vi "P2022 TB INCAR.vi"() -> ()   [LabVIEW 2013]
doc: "Use this template to build a producer/consumer design pattern with events to produce queue items. Use this design pattern instead of the user interface event handler pattern for user interfaces when you want to execute code asynchronously in response to an event without slowing the user interface responsiveness."
uses:
  Controles/P2022 Datos Control.ctl
  Controles/P2018 Com Control.ctl
  serialBronkhorst/_s_TablaBronkhorst.ctl
  Controles/P2018 Arduino Control.ctl
  Controles/Functions.ctl
  Controles/User Event Data.ctl
  Controles/Data Type.ctl
  Controles/Change Control.ctl
  Controles/PassedVars.ctl
  P2022 TB INCAR GLOBALES.vi
panel:
  out "ESTADO":T1
  out "SP_EXTRA":dbl format="%.1f"
  out "mst0":i32
  out "mst1":i32
  in  "Tab Control":T2(tab)
  out "String1f":string
  out "String2f":string
  out "String3f":string
  out "String4f":string
  out "FLUJO8":dbl caption="ln/h" format="%.2f"
  out "FLUJO7":dbl caption="ln/h" format="%.2f"
  out "FLUJO6":dbl caption="ln/h" format="%.2f"
  out "FLUJO5":dbl caption="ln/h" format="%.2f"
  out "Lvalve":bool
  out "Lflujo4":bool
  out "Lflujo3":bool
  out "Lflujo2":bool
  out "Lflujo1":bool
  in  "Modulo":u32=1 max=1000 step=1
  in  "Comments":string="Añade aqui los comentarios...... y pincha fuera (sin teclear ENTER)"
  out "TEMP_EXTRA":dbl format="%.1f"
  out "TEMP_CINTA":dbl format="%.1f"
  out "SP_CINTA":dbl format="%.1f"
  out "TEMP_INF":dbl format="%.1f"
  out "SP_TINF":dbl format="%.1f"
  out "TEMP_SUP":dbl format="%.1f"
  out "SP_TSUP":dbl format="%.1f"
  out "TIEMPO(min)":dbl format="%.2f"
  out "PESO(mg)":dbl format="%.1f"
  out "TEMPERATURA(C)":dbl format="%.1f"
  out "FLUJO4":dbl caption="ln/h" format="%.2f"
  out "FLUJO3":dbl caption="ln/h" format="%.2f"
  out "FLUJO2":dbl caption="ln/h" format="%.2f"
  out "FLUJO1":dbl caption="g/h" format="%.2f"
  out "Sampling(ms)":i32
  out "Lsample":bool
  out "Estado":string
  in  "Calibrar":bool
  in  "Muestreo":bool
  in  "Temperatura":bool
  in  "Programar":bool
  in  "Fin":bool
  in  "Auto":bool
  in  "Manual":bool
  in  "Reles":bool
  in  "Flujos":bool
  in  "Parar":bool
  out "String1s":string
  out "String2s":string
  out "String3s":string
  out "String4s":string
  out "Tempex(C),":dbl format="%.1f"
  out "XY Peso":cluster{dbl[], dbl[]}[](graph)
  out "Tiempo(min),":dbl format="%.2f"
  out "Pesotb(mg),":dbl format="%.2f"
  out "Temptb(C),":dbl format="%.1f"
  out "Ttermob(C)":dbl format="%.1f"
  out "XYTemp":cluster{dbl[], dbl[]}[](graph)
  out "Tsuperior(C)":dbl format="%.1f"
  out "Tinferior(C)":dbl format="%.1f"
  out "TcintaC)":dbl format="%.1f"
  out "Textra(C)":dbl format="%.1f"
  out "XYTemPes":cluster{dbl[], dbl[]}(graph)
  out "Temptb(C)_":dbl format="%.1f"
  out "Pesotb(mg)_":dbl format="%.2f"
  out "Flujo8.":dbl format="%.2f"
  out "Flujo7.":dbl format="%.2f"
  out "Flujo6.":dbl format="%.2f"
  out "Flujo5.":dbl format="%.2f"
  out "XYFlows":cluster{dbl[], dbl[]}[](graph)
  out "Flujo4.":dbl format="%.2f"
  out "Flujo3.":dbl format="%.2f"
  out "Flujo2.":dbl format="%.2f"
  out "Flujo1.":dbl format="%.2f"
  in  "Completa":i32(listbox)
  in  "Secuencia":bool
  in  "Reducida":i32(listbox)
  in  "Pausa":bool
  in  "Saltar":bool
  in  "Max_t (s)":dbl=900.0 min=0.0 max=999.9 step=0.1 format="%.1f"
  in  "Delta_t (s)":dbl=60.0 min=0.0 max=999.9 step=0.1 format="%.1f"
  in  "Delta_T (C)":dbl=1.0 min=0.0 max=999.9 step=0.1 format="%.1f"
  out "PASOS":string[](array[string])
  out "FLOWBUS MassFlowDevs":T3
  out "SERIAL MassFlowDevs":T3
  out "Datos":T4 {"fFSET4" format="%#.6f"; "fFSET3" format="%#.6f"; "fFSET2" format="%#.6f"; "fFSET1" format="%#.6f"; "fFLUJO4" format="%#.6f"; "fFLUJO2" format="%#.6f"; "fFLUJO1" format="%#.6f"; "fFLUJO3" format="%#.6f"; "T_EXTRA" format="%#.6f"; "TSET_EXTRA" format="%#.6f"; "T_CINTA" format="%#.6f"; "TSET_CINTA" format="%#.6f"; "sFSET4" format="%#.6f"; "POSICION" format="%#.6f"; "TEMP_SUP" format="%#.6f"; "TSET_SUP" format="%#.6f"; "PESO_TB" format="%#.6f"; "TEMP_TB" format="%#.6f"; "TEMP_INF" format="%#.6f"; "sFSET3" format="%#.6f"; "sFSET2" format="%#.6f"; "sFSET1" format="%#.6f"; "V_VAPOR" format="%#.6f"; "sFLUJO4" format="%#.6f"; "sFLUJO2" format="%#.6f"; "sFLUJO1" format="%#.6f"; "TSET_INF" format="%#.6f"; "TIEMPO" format="%#.6f"; "sFLUJO3" format="%#.6f"}
  out "error out":errorcluster
  out "Comunicaciones":T5={"Flujo_1"="ASRL6::INSTR", "Brk1"=FALSE, "Flujo_2"="ASRL6::INSTR", "Brk2"=FALSE, "Flujo_3"="ASRL6::INSTR", "Brk3"=FALSE, "Flujo_4"="ASRL6::INSTR", "Brk4"=FALSE, "Eurothe"="ASRL6::INSTR", "Eurot"=FALSE, "Balanza"="ASRL6::INSTR", "Bal"=FALSE, "eValPos"="ASRL6::INSTR", "eVal"=FALSE, "flowbus"="ASRL6::INSTR", "fb"=FALSE}
  out "PESO":string
  out "TEMPERATURA":string
  out "Array":dbl[][](array[numeric])
  in  "Secuencia":string[](array[string])
  # "INCAR  TB \nEnero 2023 Ver2.3.1"
  # "a-sslcdms 01/2023"
  # "Termobalanza      ___________________________________"
  # "Horno y cinta"
  # "Temperatura extra"
  # "Termobalanza"
  # "Termobalanza      ___________________________"
  # "SERIE                          Controladores de flujo                     FLOWBUS"
  # "Condiciones de estabilidad en temperatura"
  # "Maxima variación \nde temperatura"
  # "en este intervalo \nde tiempo."
  # "Maximo tiempo posible \nsin alcanzar estabilidad"
  # "TERMOBALANZA"
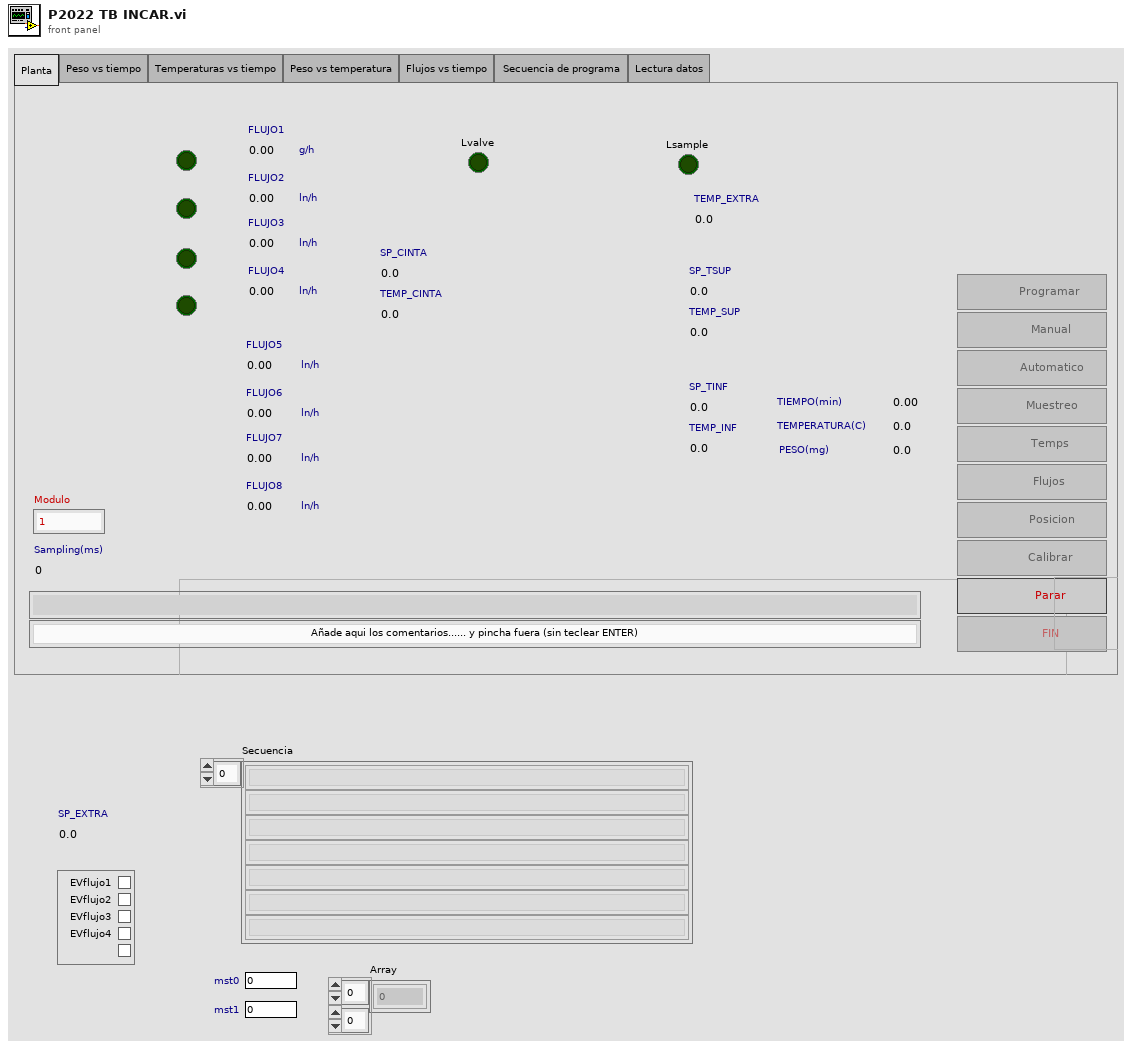
[diagram p1: front panel]
types:
  T1 = typedef "P2018 Arduino Control.ctl" = cluster{"EVflujo1":bool, "EVflujo2":bool, "EVflujo3":bool, "EVflujo4":bool, "Evalve":bool}
  T2 = enum32{"Planta", "Peso vs tiempo", "Temperaturas vs tiempo", "Peso vs temperatura", "Flujos vs tiempo", "Secuencia de programa ", "Lectura datos"}
  T3 = typedef "_s_TablaBronkhorst.ctl" = string[][]
  T4 = typedef "P2022 Datos Control.ctl" = cluster{"TIEMPO":dbl, "sFSET1":dbl, "sFLUJO1":dbl, "sFSET2":dbl, "sFLUJO2":dbl, "sFSET3":dbl, "sFLUJO3":dbl, "sFSET4":dbl, "sFLUJO4":dbl, "TSET_SUP":dbl, "TEMP_SUP":dbl, "TSET_INF":dbl, "TEMP_INF":dbl, "TSET_CINTA":dbl, "T_CINTA":dbl, "TSET_EXTRA":dbl, "T_EXTRA":dbl, "TEMP_TB":dbl, "PESO_TB":dbl, "POSICION":dbl, "V_VAPOR":dbl, "fFSET1":dbl, "fFLUJO1":dbl, "fFSET2":dbl, "fFLUJO2":dbl, "fFSET3":dbl, "fFLUJO3":dbl, "fFSET4":dbl, "fFLUJO4":dbl}
  T5 = typedef "P2018 Com Control.ctl" = cluster{"Flujo_1":refnum<visa-resource-name>, "Brk1":bool, "Flujo_2":refnum<visa-resource-name>, "Brk2":bool, "Flujo_3":refnum<visa-resource-name>, "Brk3":bool, "Flujo_4":refnum<visa-resource-name>, "Brk4":bool, "Eurothe":refnum<visa-resource-name>, "Eurot":bool, "Balanza":refnum<visa-resource-name>, "Bal":bool, "eValPos":refnum<visa-resource-name>, "eVal":bool, "flowbus":refnum<visa-resource-name>, "fb":bool}
  T6 = enum32{"Planta", "Peso vs tiempo", "Temperaturas vs tiempo", "Peso vs temperatura", "Flujos vs tiempo", "Secuencia de programa "}
  T7 = typedef "User Event Data.ctl" = cluster{"Data Type":T8, "Data":variant}
  T8 = typedef "Data Type.ctl" = enum16{"Init FP", "En/Dis FP Ctls", "Update FP", "Upd Status", "Upd Seq"}
  T9 = typedef "Functions.ctl" = enum16{"Initialize", "Run Man", "Run Auto", "Stop"}
  T10 = typedef "Change Control.ctl" = enum16{"Default", "Continue", "Change Flows", "Change Valves", "Change Temp"}
  T11 = typedef "PassedVars.ctl" = dbl
  T12 = typedef "P2018 Bronkhorst Control.ctl" = cluster{"Dispositivos":T3, "NuevosSP":string[][], "Nodes":u32, "Delay(s)":dbl}
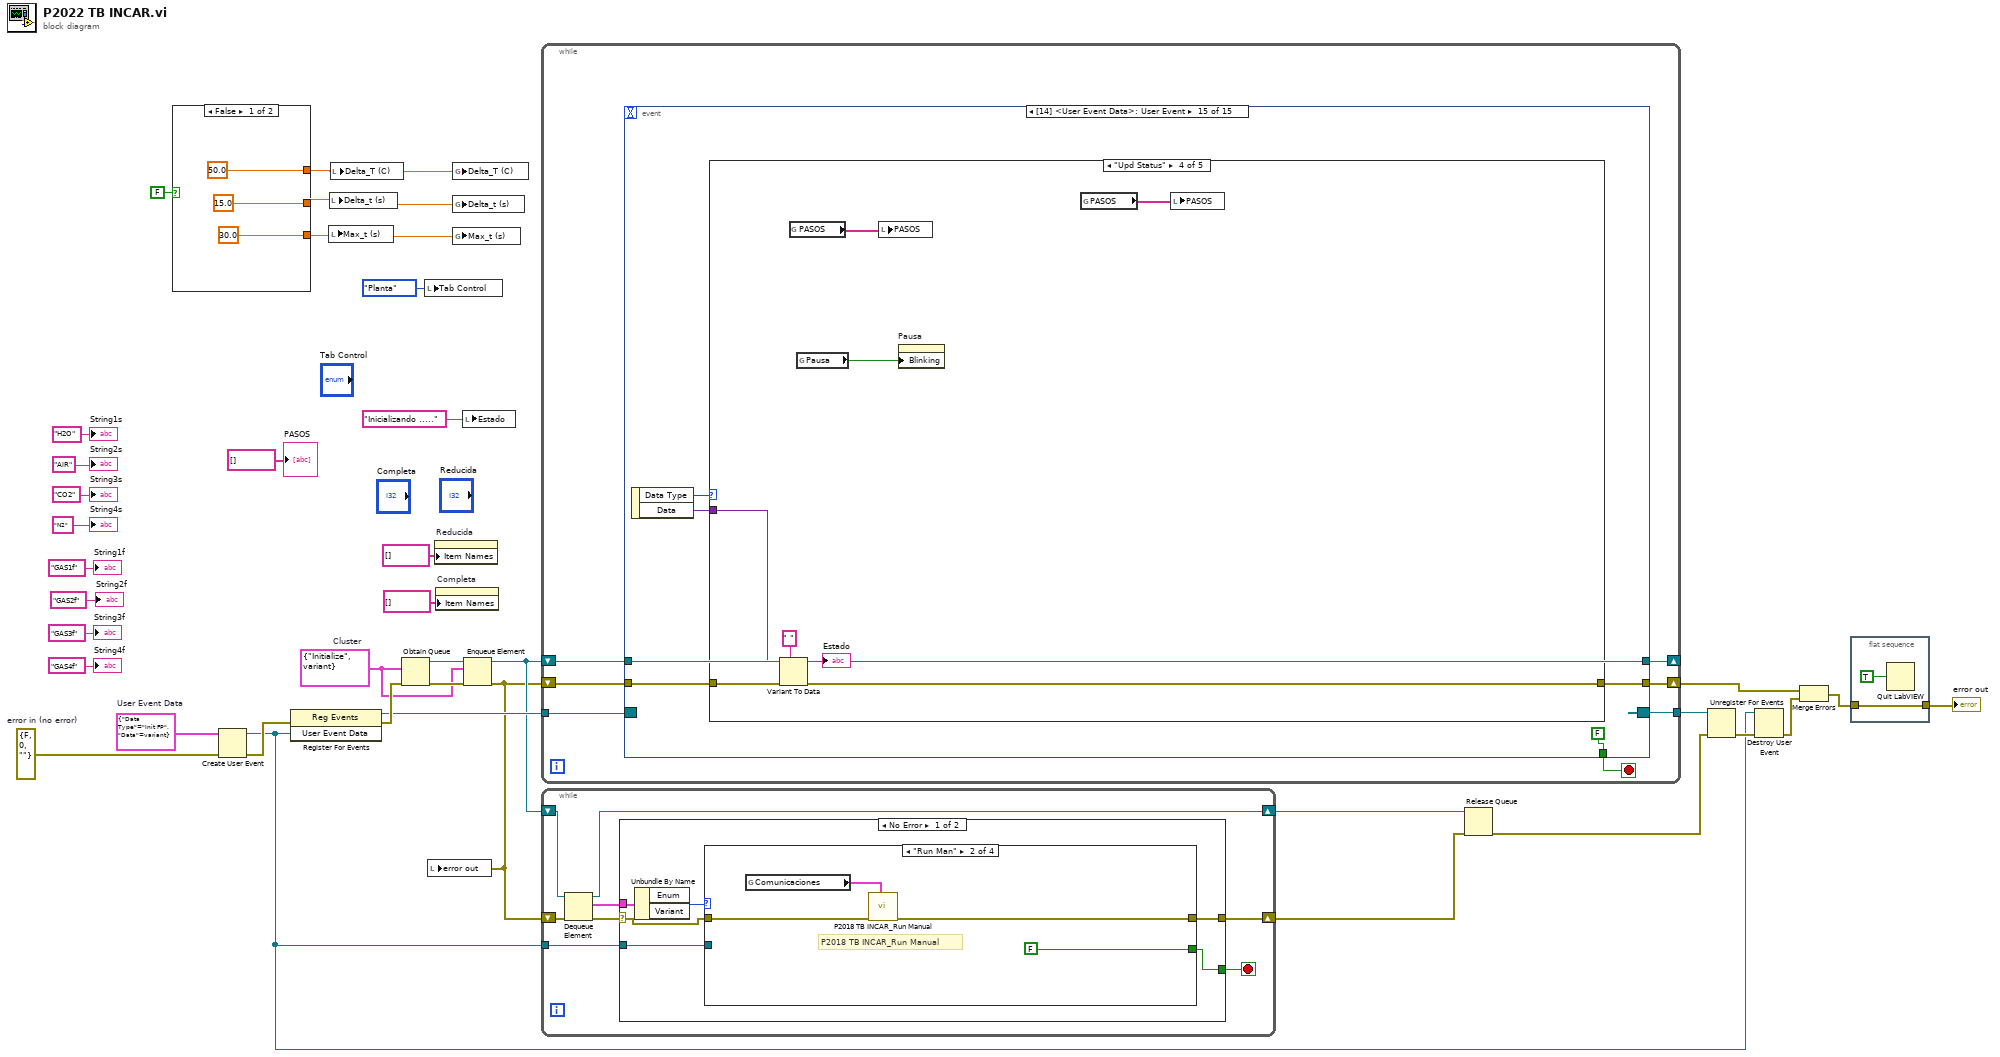
[diagram p0: block diagram]
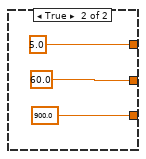
[diagram p2: hidden frame]
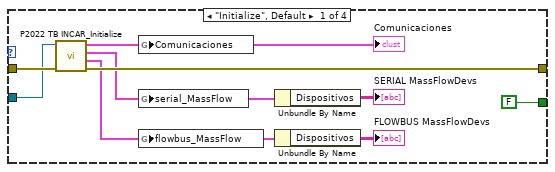
[diagram p3: hidden frame]
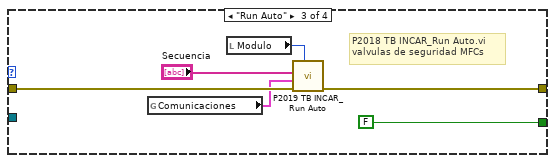
[diagram p4: hidden frame]
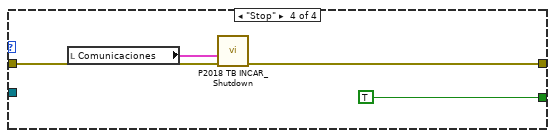
[diagram p5: hidden frame]
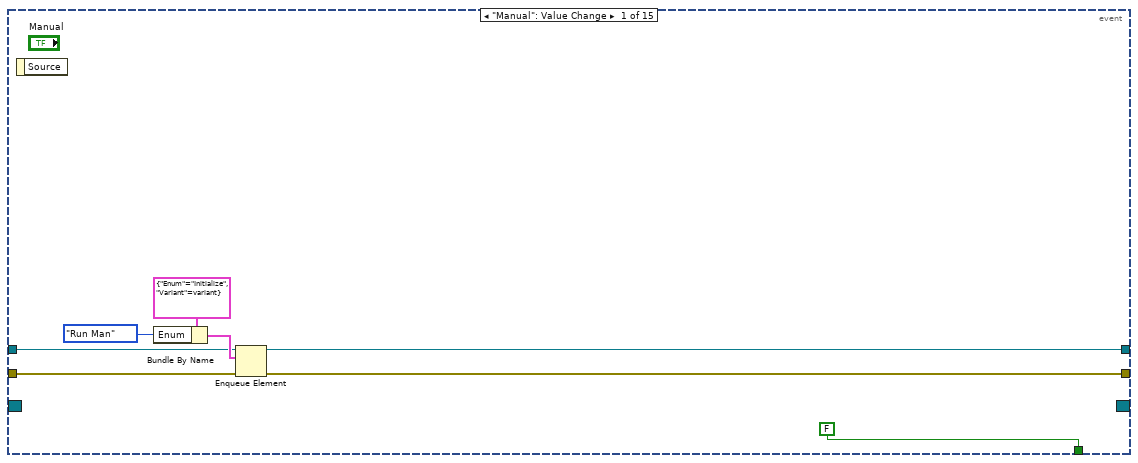
[diagram p7: hidden frame]
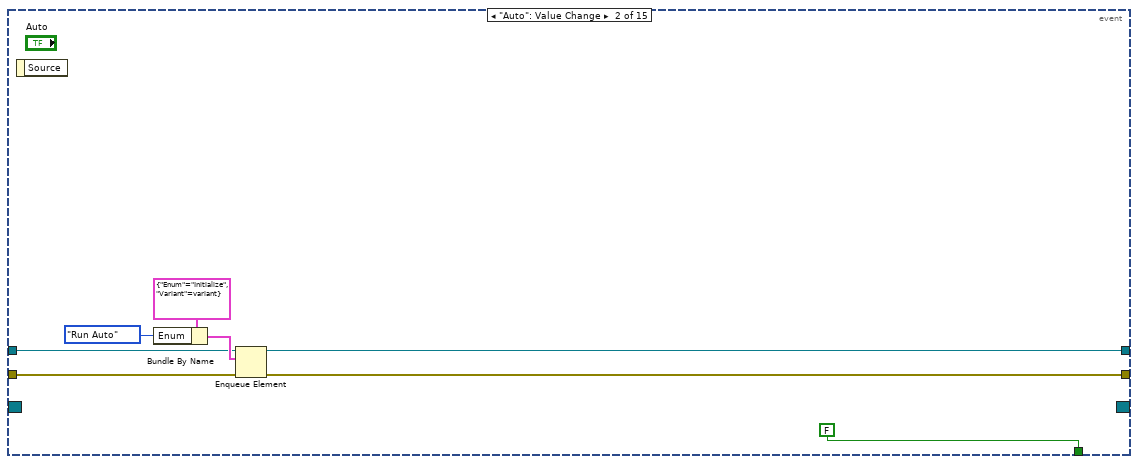
[diagram p8: hidden frame]
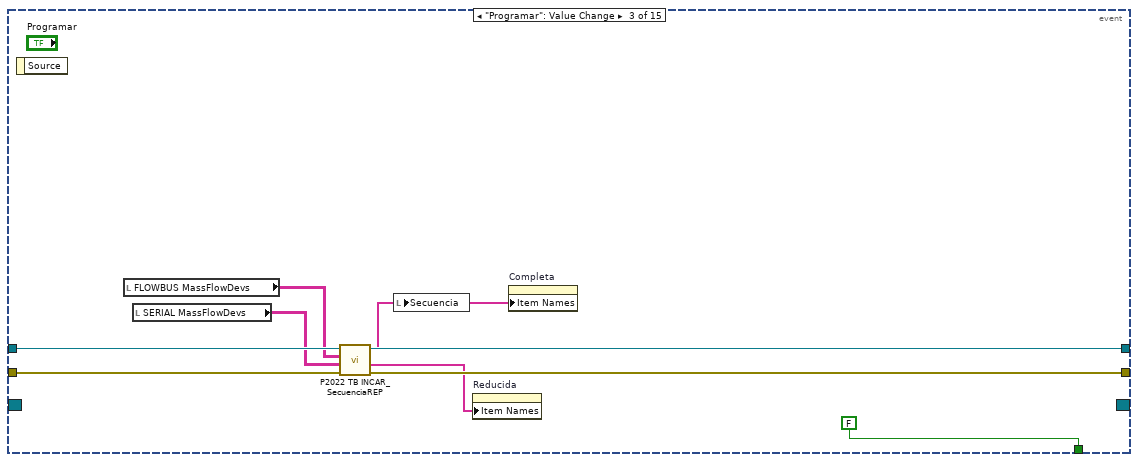
[diagram p9: hidden frame]
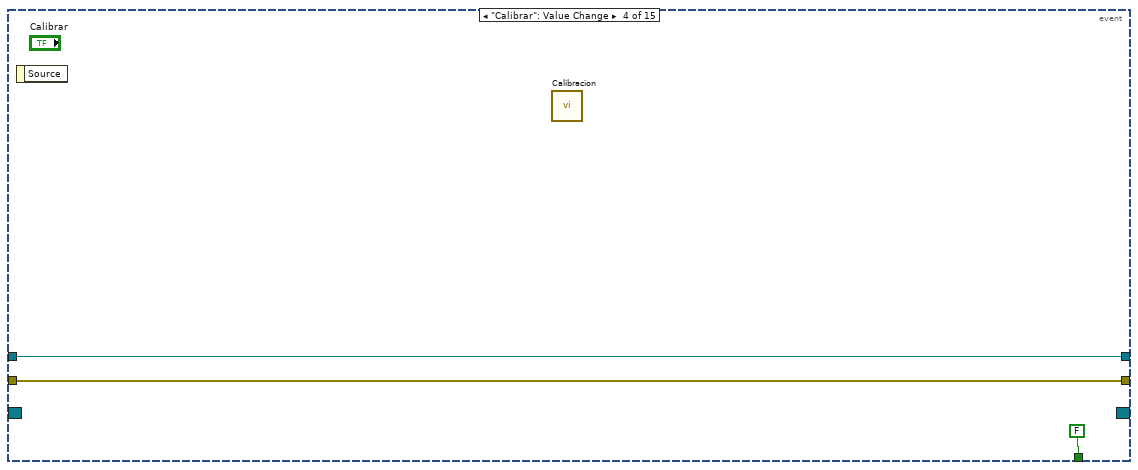
[diagram p10: hidden frame]
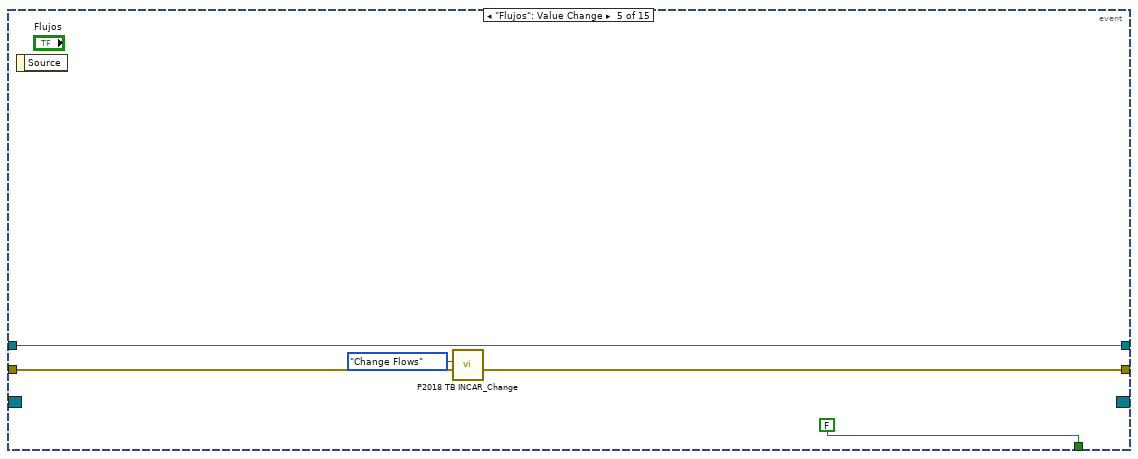
[diagram p11: hidden frame]
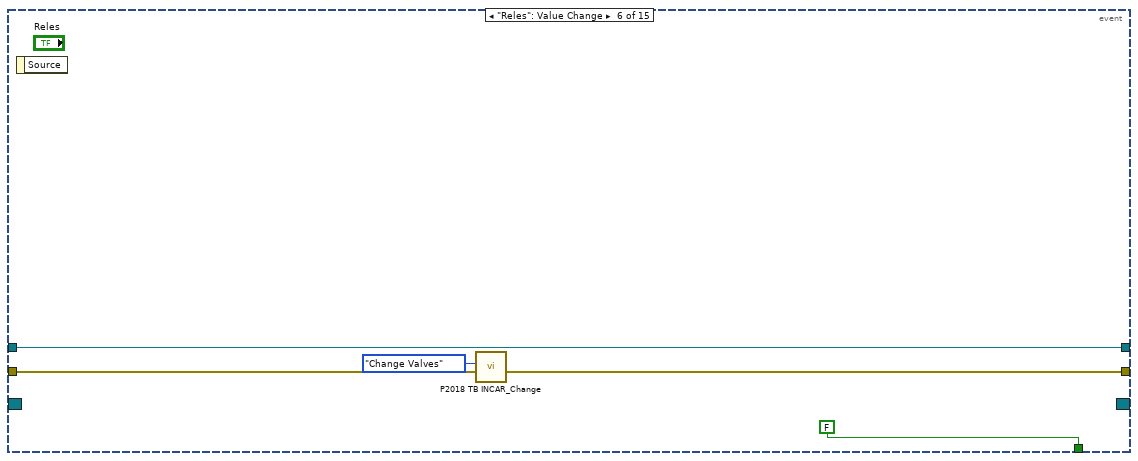
[diagram p12: hidden frame]
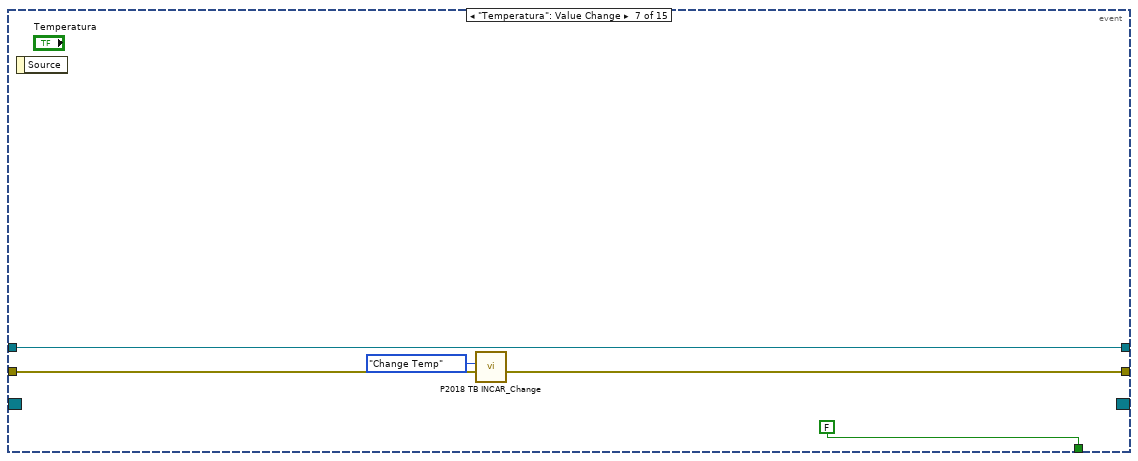
[diagram p13: hidden frame]
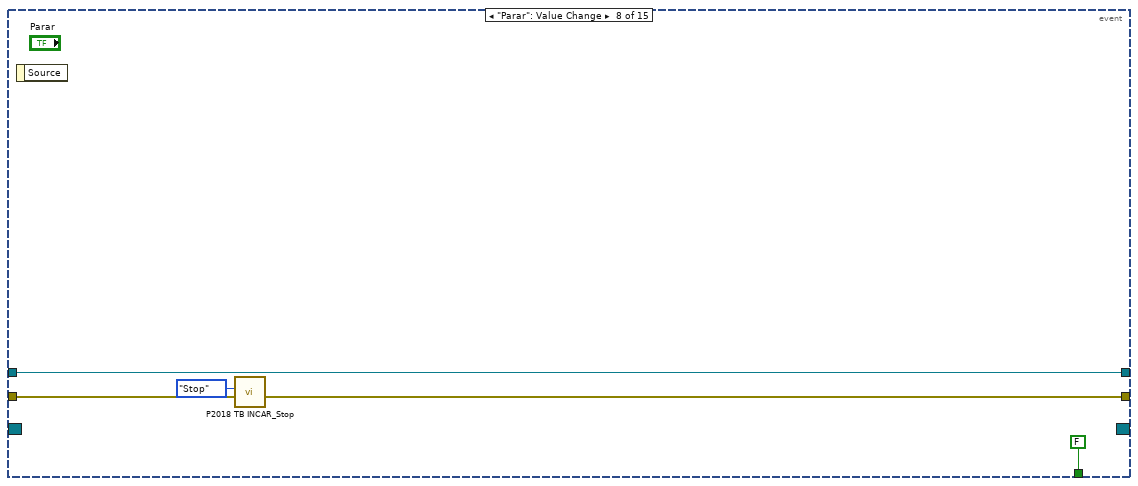
[diagram p14: hidden frame]
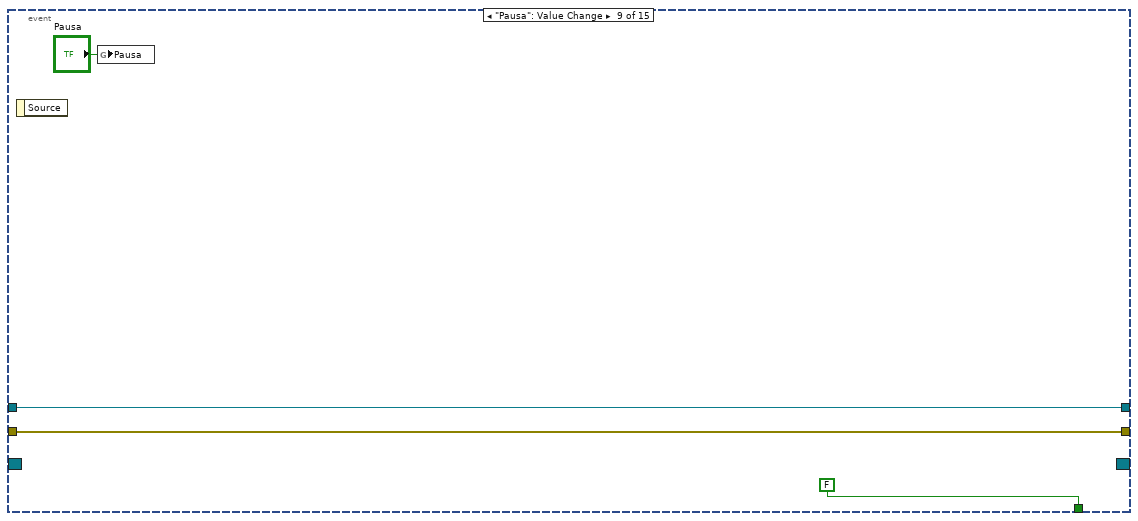
[diagram p15: hidden frame]
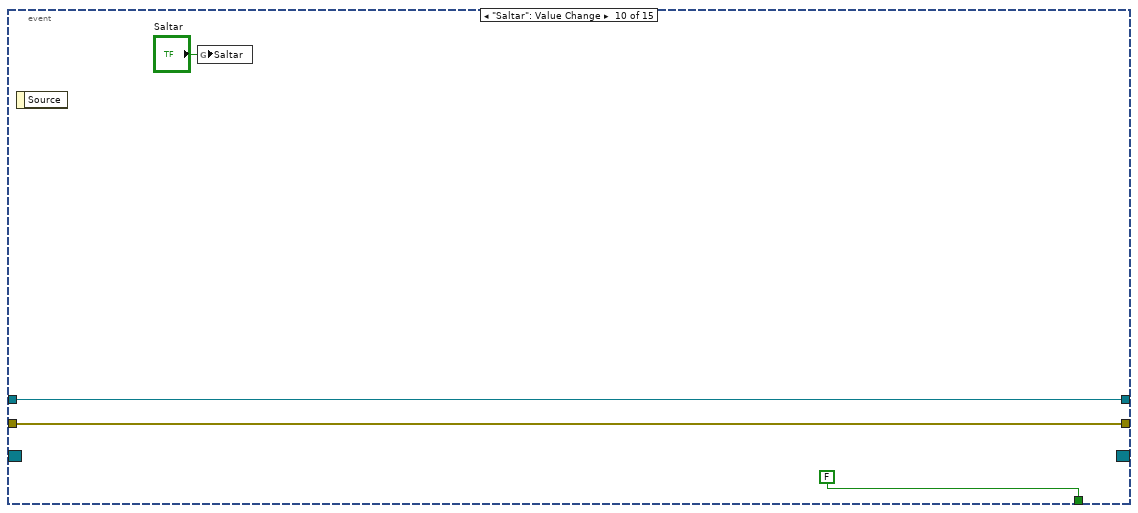
[diagram p16: hidden frame]
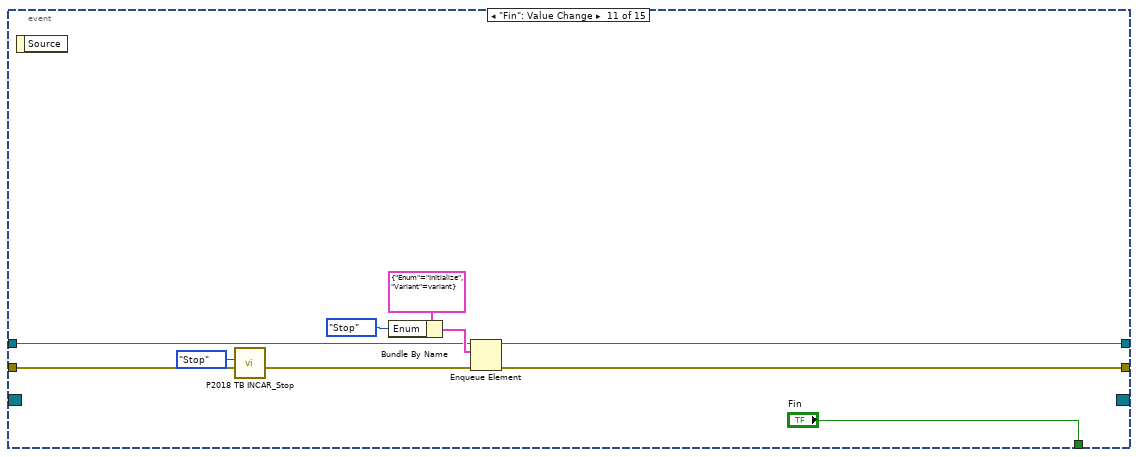
[diagram p17: hidden frame]
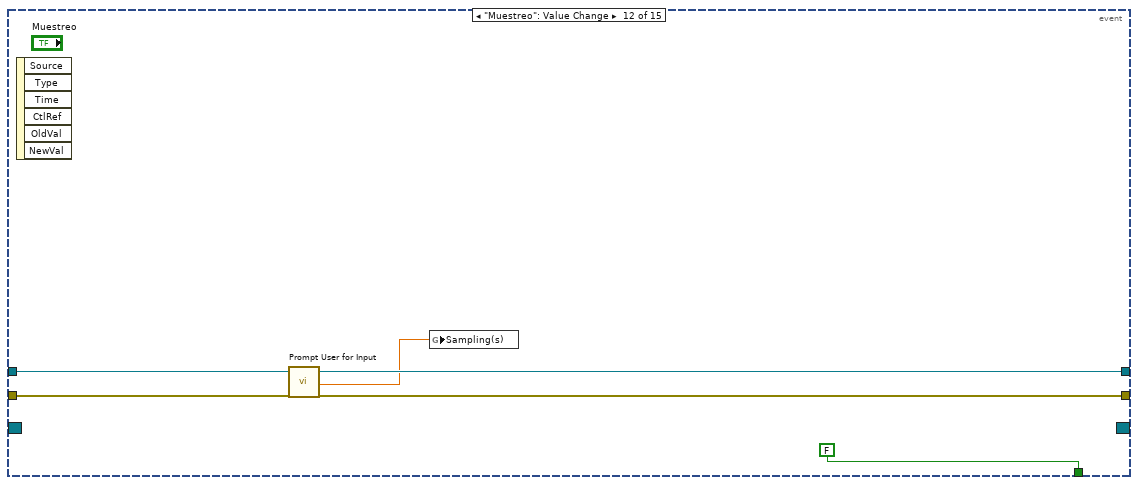
[diagram p18: hidden frame]
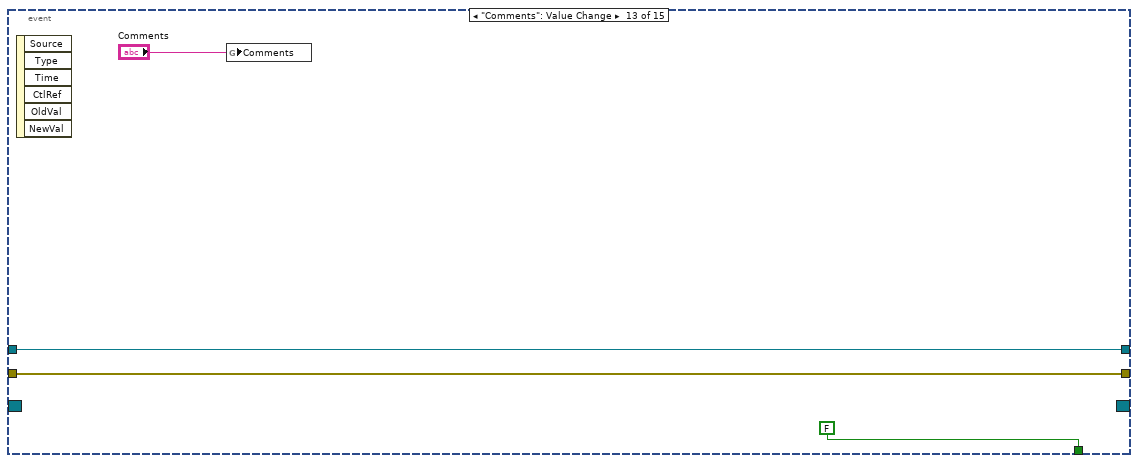
[diagram p19: hidden frame]
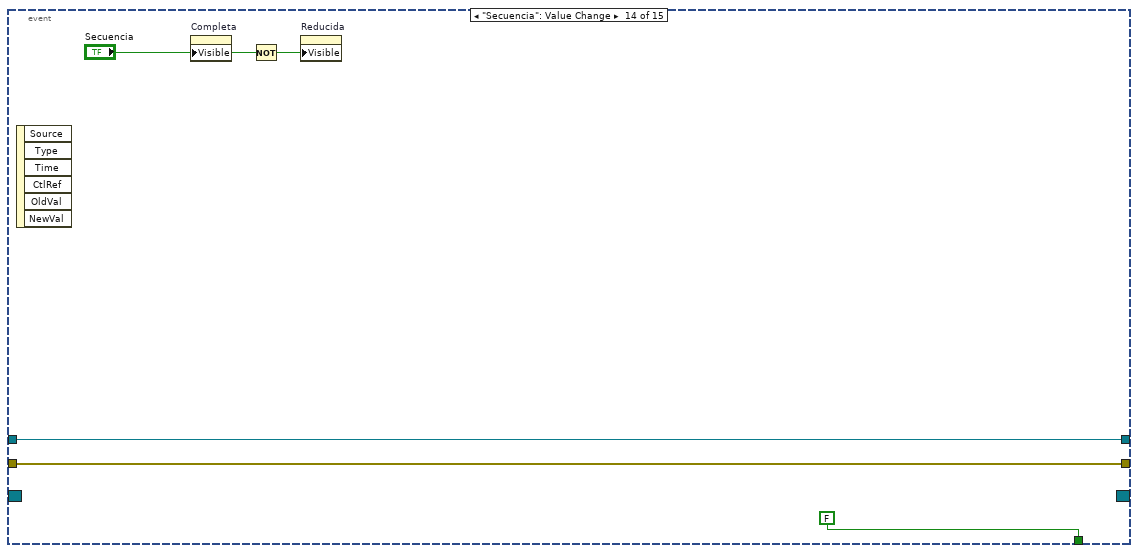
[diagram p20: hidden frame]
diagram:
  w24 = T7 {"Data Type"=enum."Init FP", "Data"=variant}  # User Event Data
  w16 = errorcluster {"status"=FALSE, "code"=0, "source"=""}  # error in (no error)
  w34 = cluster{"Enum":T9, "Variant":variant} {"Enum"=enum."Initialize", "Variant"=variant}  # Cluster
  n1 = case shown="False" FALSE {
    tunnel: [50.0 ("Delta_T (C)") 5.0 ("Delta_T (C)")] -> w14
    tunnel: [15.0 ("Delta_t (s)") 60.0 ("Delta_t (s)")] -> w13
    tunnel: [30.0 ("Max_t (s)") 900.0 ("Max_t (s)")] -> w12
    frame False {
    }
    frame True {
    }
  }
  n2 = Create User Event(user event datatype=w24, error in=w16) -> (user event=w21:refnum<user-event>, error out=w36:errorcluster)
  n3 = register-events(error in=w36, w21) -> (reference out=w26:refnum<event-registration>, error out=w37:errorcluster)  [unwired: 1 in]
  n4 = local write "Max_t (s)"(w12) -> ()
  n5 = local write "Delta_t (s)"(w13) -> ()
  n6 = local write "Delta_T (C)"(w14) -> ()
  n7 = Obtain Queue(element data type=w34, error in (no error)=w37) -> (queue out=w33:refnum<queue>, error out=w35:errorcluster)  [unwired: 3 in, 1 out]
  n8 = local write "Tab Control"(T6."Planta" ("Tab Control")) -> ()
  n9 = property on="Reducida" class="LstBox (strict)"("Item Names"=string[] []) -> ()  [unwired: 2 in, 2 out]
  n10 = property on="Completa" class="LstBox (strict)"("Item Names"=string[] []) -> ()  [unwired: 2 in, 2 out]
  n11 = global write "P2022 TB INCAR GLOBALES.vi" "Delta_T (C)"(w14) -> ()
  n12 = global write "P2022 TB INCAR GLOBALES.vi" "Delta_t (s)"(w13) -> ()
  n13 = global write "P2022 TB INCAR GLOBALES.vi" "Max_t (s)"(w12) -> ()
  n14 = local write "Estado"("Inicializando ....." ("String")) -> ()
  n15 = Enqueue Element(queue=w33, element=w34, error in (no error)=w35) -> (queue out=w23:refnum<queue>, error out=w22:errorcluster)  [unwired: 1 in, 1 out]
  n16 = local write "error out"(w22) -> ()
  n17 = while {
    shift-right: [w44] -> w29
    shift-left: w22 -> [w48]
    shift-right: [w49] -> _
    shift-left: w23 -> [w50]
    tunnel: w26 -> [w46]
    tunnel: [w45] -> w25
    stop <- w47 stop-if-true
    n18 = event shown="[14] <User Event Data>: User Event" {
      selector: w46 -> [_ _ _ _ _ _ _ _ _ _ _ _ _ _ _]
      dyn-events: [_ _ _ _ _ _ _ _ _ _ _ _ _ _ _] -> w45
      timeout: _ -> [_ _ _ _ _ _ _ _ _ _ _ _ _ _ _]
      tunnel: w50 -> [w53 w61 w73 w76 w80 w84 w89 w94 w100 w104 w110 w120 w124 w129 w131]
      tunnel: [w54 w62 w73 w76 w80 w84 w89 w94 w100 w104 w111 w120 w124 w129 w131] -> w49
      tunnel: w48 -> [w52 w60 w72 w75 w79 w86 w91 w96 w98 w102 w108 w118 w121 w125 w133]
      tunnel: [w55 w63 w71 w75 w81 w85 w90 w93 w98 w102 w112 w117 w121 w125 w132] -> w44
      tunnel: [FALSE ("Parar") FALSE ("Parar") FALSE ("Parar") FALSE ("Parar") FALSE ("Parar") FALSE ("Parar") FALSE ("Parar") FALSE ("Parar") FALSE ("Parar") FALSE ("Parar") "Fin" FALSE ("Parar") FALSE ("Parar") FALSE ("Parar") FALSE ("Parar")] -> w47
      event "Manual": Value Change {
        n19 = event-data() -> ()  [unwired: 1 in, 1 out]
        n20 = Bundle By Name(cluster=cluster{"Enum":T9, "Variant":variant} {"Enum"=enum."Initialize", "Variant"=variant} ("Cluster"), "Enum"=Functions."Run Man") -> (w56:cluster{"Enum":T9, "Variant":variant})
        n21 = Enqueue Element(queue=w53, element=w56, error in (no error)=w52) -> (queue out=w54:refnum<queue>, error out=w55:errorcluster)  [unwired: 1 in, 1 out]
      }
      event "Auto": Value Change {
        n22 = event-data() -> ()  [unwired: 1 in, 1 out]
        n23 = Bundle By Name(cluster=cluster{"Enum":T9, "Variant":variant} {"Enum"=enum."Initialize", "Variant"=variant} ("Cluster"), "Enum"=Functions."Run Auto") -> (w64:cluster{"Enum":T9, "Variant":variant})
        n24 = Enqueue Element(queue=w61, element=w64, error in (no error)=w60) -> (queue out=w62:refnum<queue>, error out=w63:errorcluster)  [unwired: 1 in, 1 out]
      }
      event "Programar": Value Change {
        n25 = event-data() -> ()  [unwired: 1 in, 1 out]
        n26 = local read "FLOWBUS MassFlowDevs"() -> (w67:T3)
        n27 = local read "SERIAL MassFlowDevs"() -> (w70:T3)
        n28 = call "P2022 TB INCAR_SecuenciaREP.vi"("error in (no error)"=w72, "SERIAL MassFlowDevs"=w70, "FLOWBUS MassFlowDevs"=w67) -> ("error out"=w71:errorcluster, "Secuencia"=w68:string[], "Secuciclos"=w69:string[])  [unwired: 4 in, 2 out]
        n29 = local write "Secuencia"(w69) -> ()
        n30 = property on="Reducida" class="LstBox (strict)"("Item Names"=w68) -> ()  [unwired: 2 in, 2 out]
        n31 = property on="Completa" class="LstBox (strict)"("Item Names"=w69) -> ()  [unwired: 2 in, 2 out]
      }
      event "Calibrar": Value Change {
        n32 = event-data() -> ()  [unwired: 1 in, 1 out]
        n33 = call "Calibracion.vi"() -> ()  [unwired: 1 in]
      }
      event "Flujos": Value Change {
        n34 = event-data() -> ()  [unwired: 1 in, 1 out]
        n35 = call "P2018 TB INCAR_Change.vi"("error in (no error)"=w79, "Change"=Change_Control."Change Flows") -> ("error out"=w81:errorcluster)  [unwired: 8 in, 1 out]
      }
      event "Reles": Value Change {
        n36 = event-data() -> ()  [unwired: 1 in, 1 out]
        n37 = call "P2018 TB INCAR_Change.vi"("error in (no error)"=w86, "Change"=Change_Control."Change Valves") -> ("error out"=w85:errorcluster)  [unwired: 8 in, 1 out]
      }
      event "Temperatura": Value Change {
        n38 = event-data() -> ()  [unwired: 1 in, 1 out]
        n39 = call "P2018 TB INCAR_Change.vi"("error in (no error)"=w91, "Change"=Change_Control."Change Temp") -> ("error out"=w90:errorcluster)  [unwired: 8 in, 1 out]
      }
      event "Parar": Value Change {
        n40 = event-data() -> ()  [unwired: 1 in, 1 out]
        n41 = call "P2018 TB INCAR_Stop.vi"("error in (no error)"=w96, "Stop"=enum16{"Continue", "Stop", "Default"}."Stop") -> ("error out"=w93:errorcluster)  [unwired: 8 in, 1 out]
      }
      event "Pausa": Value Change {
        n42 = event-data() -> ()  [unwired: 1 in, 1 out]
        n43 = global write "P2022 TB INCAR GLOBALES.vi" "Pausa"("Pausa") -> ()
      }
      event "Saltar": Value Change {
        n44 = event-data() -> ()  [unwired: 1 in, 1 out]
        n45 = global write "P2022 TB INCAR GLOBALES.vi" "Saltar"("Saltar") -> ()
      }
      event "Fin": Value Change {
        n46 = event-data() -> ()  [unwired: 1 in, 1 out]
        n47 = call "P2018 TB INCAR_Stop.vi"("error in (no error)"=w108, "Stop"=enum16{"Continue", "Stop", "Default"}."Stop") -> ("error out"=w107:errorcluster)  [unwired: 8 in, 1 out]
        n48 = Bundle By Name(cluster=cluster{"Enum":T9, "Variant":variant} {"Enum"=enum."Initialize", "Variant"=variant} ("Cluster"), "Enum"=Functions."Stop") -> (w113:cluster{"Enum":T9, "Variant":variant})
        n49 = Enqueue Element(queue=w110, element=w113, error in (no error)=w107) -> (queue out=w111:refnum<queue>, error out=w112:errorcluster)  [unwired: 1 in, 1 out]
      }
      event "Muestreo": Value Change {
        n50 = event-data() -> ()  [unwired: 1 in, 6 out]
        n51 = call "Prompt User for Input"("error in (no error)"=w118) -> ("Muestreo (s)"=w116:dbl, "error out"=w117:errorcluster)  [unwired: 16 in, 1 out]
        n52 = global write "P2022 TB INCAR GLOBALES.vi" "Sampling(s)"(w116) -> ()
      }
      event "Comments": Value Change {
        n53 = event-data() -> ()  [unwired: 1 in, 6 out]
        n54 = global write "P2022 TB INCAR GLOBALES.vi" "Comments"("Comments") -> ()
      }
      event "Secuencia": Value Change {
        n55 = event-data() -> ()  [unwired: 1 in, 6 out]
        n56 = property on="Completa" class="LstBox (strict)"("Visible"="Secuencia") -> ()  [unwired: 2 in, 2 out]
        n57 = Not(x="Secuencia") -> (.not. x?=w127:bool)
        n58 = property on="Reducida" class="LstBox (strict)"("Visible"=w127) -> ()  [unwired: 2 in, 2 out]
      }
      event User Event {
        n59 = event-data() -> ("Data Type"=w135:T8, "Data"=w134:variant)  [unwired: 1 in]
        n60 = case shown="\"Upd Status\"" w135 {
          tunnel: w134 -> [_ w148 w282 w295 w300]
          tunnel: w133 -> [w144 w151 w283 w294 w302]
          tunnel: [w144 w150 w263 w293 w301] -> w132
          frame "Init FP", Default {
            w140 = cluster{dbl[], dbl[]}[] [] ("XYFlows")
            n61 = global read "P2022 TB INCAR GLOBALES.vi" "Arduino"() -> (w137:T1)
            n62 = local write "ESTADO"(w137) -> ()
            n63 = local write "Modulo"(u32 1 ("ModuloIN")) -> ()
            n64 = local write "XYFlows"(w140) -> ()
            n65 = local write "XYTemp"(w140) -> ()
            n66 = local write "Estado"("Listo para comenzar" ("String")) -> ()
            n67 = local write "XY Peso"(w140) -> ()
            n68 = global write "P2022 TB INCAR GLOBALES.vi" "Sampling(s)"(T11 10.0 ("Lectura")) -> ()
            n69 = local write "XYTemPes"(cluster{dbl[], dbl[]} {[], []} ("XY Peso")) -> ()
            n70 = property on="Datos" class="Clust (strict)"("Value"=T4 {"TIEMPO"=0.0, "sFSET1"=0.0, "sFLUJO1"=0.0, "sFSET2"=0.0, "sFLUJO2"=0.0, "sFSET3"=0.0, "sFLUJO3"=0.0, "sFSET4"=0.0, "sFLUJO4"=0.0, "TSET_SUP"=0.0, "TEMP_SUP"=0.0, "TSET_INF"=0.0, "TEMP_INF"=0.0, "TSET_CINTA"=0.0, "T_CINTA"=0.0, "TSET_EXTRA"=0.0, "T_EXTRA"=0.0, "TEMP_TB"=0.0, "PESO_TB"=0.0, "POSICION"=0.0, "V_VAPOR"=0.0, "fFSET1"=0.0, "fFLUJO1"=0.0, "fFSET2"=0.0, "fFLUJO2"=0.0, "fFSET3"=0.0, "fFLUJO3"=0.0, "fFSET4"=0.0, "fFLUJO4"=0.0} ("Datos")) -> ()  [unwired: 2 in, 2 out]
            "Array" <- dbl[][] [] ("Array")
          }
          frame "En/Dis FP Ctls" {
            n71 = Variant To Data(error in=w151, type=0, Variant=w148) -> (data=w147:i32, error out=w150:errorcluster)
            n72 = property on="Saltar" class="Bool"("Disabled"=u8 2) -> ()  [unwired: 2 in, 2 out]
            n73 = property on="Pausa" class="Bool (strict)"("Disabled"=u8 2) -> ()  [unwired: 2 in, 2 out]
            n74 = case shown="0, Default" w147 {
              frame 0, Default {
                # "Programa en pausa"
                n75 = property on="Reles" class="Bool"("Disabled"=u8 2) -> ()  [unwired: 2 in, 2 out]
                n76 = property on="Flujos" class="Bool"("Disabled"=u8 2) -> ()  [unwired: 2 in, 2 out]
                n77 = property on="Programar" class="Bool"("Disabled"=u8 0) -> ()  [unwired: 2 in, 2 out]
                n78 = property on="Saltar" class="Bool"("Disabled"=u8 2) -> ()  [unwired: 2 in, 2 out]
                n79 = property on="Pausa" class="Bool (strict)"("Disabled"=u8 2) -> ()  [unwired: 2 in, 2 out]
                n80 = property on="Temperatura" class="Bool"("Disabled"=u8 2) -> ()  [unwired: 2 in, 2 out]
                n81 = property on="Muestreo" class="Bool"("Disabled"=u8 2) -> ()  [unwired: 2 in, 2 out]
                n82 = property on="Parar" class="Bool"("Disabled"=u8 2) -> ()  [unwired: 2 in, 2 out]
                n83 = property on="Manual" class="Bool"("Disabled"=u8 0) -> ()  [unwired: 2 in, 2 out]
                n84 = property on="Auto" class="Bool"("Disabled"=u8 0) -> ()  [unwired: 2 in, 2 out]
                n85 = property on="Fin" class="Bool"("Disabled"=u8 0) -> ()  [unwired: 2 in, 2 out]
                n86 = property on="Calibrar" class="Bool"("Disabled"=u8 0) -> ()  [unwired: 2 in, 2 out]
              }
              frame 1 {
                # "Programa en manual"
                n87 = property on="Reles" class="Bool"("Disabled"=u8 0) -> ()  [unwired: 2 in, 2 out]
                n88 = property on="Flujos" class="Bool"("Disabled"=u8 0) -> ()  [unwired: 2 in, 2 out]
                n89 = property on="Programar" class="Bool"("Disabled"=u8 2) -> ()  [unwired: 2 in, 2 out]
                n90 = property on="Temperatura" class="Bool"("Disabled"=u8 0) -> ()  [unwired: 2 in, 2 out]
                n91 = property on="Muestreo" class="Bool"("Disabled"=u8 0) -> ()  [unwired: 2 in, 2 out]
                n92 = property on="Saltar" class="Bool"("Disabled"=u8 2) -> ()  [unwired: 2 in, 2 out]
                n93 = property on="Pausa" class="Bool (strict)"("Disabled"=u8 2) -> ()  [unwired: 2 in, 2 out]
                n94 = property on="Parar" class="Bool"("Disabled"=u8 0) -> ()  [unwired: 2 in, 2 out]
                n95 = property on="Manual" class="Bool"("Disabled"=u8 2) -> ()  [unwired: 2 in, 2 out]
                n96 = property on="Auto" class="Bool"("Disabled"=u8 2) -> ()  [unwired: 2 in, 2 out]
                n97 = property on="Fin" class="Bool"("Disabled"=u8 2) -> ()  [unwired: 2 in, 2 out]
                n98 = property on="Calibrar" class="Bool"("Disabled"=u8 2) -> ()  [unwired: 2 in, 2 out]
              }
              frame 2 {
                # "Programa en automatico"
                n99 = property on="Reles" class="Bool"("Disabled"=u8 2) -> ()  [unwired: 2 in, 2 out]
                n100 = property on="Flujos" class="Bool"("Disabled"=u8 2) -> ()  [unwired: 2 in, 2 out]
                n101 = property on="Programar" class="Bool"("Disabled"=u8 2) -> ()  [unwired: 2 in, 2 out]
                n102 = property on="Temperatura" class="Bool"("Disabled"=u8 2) -> ()  [unwired: 2 in, 2 out]
                n103 = property on="Muestreo" class="Bool"("Disabled"=u8 2) -> ()  [unwired: 2 in, 2 out]
                n104 = property on="Saltar" class="Bool"("Disabled"=u8 0) -> ()  [unwired: 2 in, 2 out]
                n105 = property on="Pausa" class="Bool (strict)"("Disabled"=u8 0) -> ()  [unwired: 2 in, 2 out]
                n106 = property on="Parar" class="Bool"("Disabled"=u8 0) -> ()  [unwired: 2 in, 2 out]
                n107 = property on="Manual" class="Bool"("Disabled"=u8 2) -> ()  [unwired: 2 in, 2 out]
                n108 = property on="Auto" class="Bool"("Disabled"=u8 2) -> ()  [unwired: 2 in, 2 out]
                n109 = property on="Fin" class="Bool"("Disabled"=u8 2) -> ()  [unwired: 2 in, 2 out]
                n110 = property on="Calibrar" class="Bool"("Disabled"=u8 2) -> ()  [unwired: 2 in, 2 out]
              }
            }
          }
          frame "Update FP" {
            # "Planta general"
            n111 = local read "Lsample"() -> (w255:bool)
            n112 = local read "Datos"() -> (w274:T4)
            n113 = Variant To Data(error in=w283, type=w274, Variant=w282) -> (data=w256:T4, error out=w263:errorcluster)
            "Datos" <- w256
            n114 = Not(x=w255) -> (.not. x?=→"Lsample":bool)
            n115 = local read "Array"() -> (w281:dbl[][])
            n116 = Unbundle By Name(w256) -> ("TIEMPO"=→"Tiempo(min)," →"TIEMPO(min)":dbl, "TSET_SUP"=→"SP_TSUP":dbl, "TEMP_SUP"=→"Tsuperior(C)" →"TEMP_SUP":dbl, "TSET_INF"=→"SP_TINF":dbl, "TEMP_INF"=→"Tinferior(C)" →"TEMP_INF":dbl, "TEMP_TB"=→"Ttermob(C)" →"Temptb(C)_" →"Temptb(C)," →"TEMPERATURA(C)":dbl, "PESO_TB"=→"Pesotb(mg)_" →"Pesotb(mg)," →"PESO(mg)":dbl, "sFLUJO1"=→"Flujo1." →"FLUJO1":dbl, "sFLUJO2"=→"Flujo2." →"FLUJO2":dbl, "sFLUJO3"=→"Flujo3." →"FLUJO3":dbl, "sFLUJO4"=→"Flujo4." →"FLUJO4":dbl, "TSET_CINTA"=→"SP_CINTA":dbl, "T_CINTA"=→"TcintaC)" →"TEMP_CINTA":dbl, "TSET_EXTRA"=→"SP_EXTRA":dbl, "T_EXTRA"=→"Textra(C)" →"TEMP_EXTRA" →"Tempex(C),":dbl, "fFLUJO1"=→"Flujo5." →"FLUJO5":dbl, "fFLUJO2"=→"Flujo6." →"FLUJO6":dbl, "fFLUJO3"=→"Flujo7." →"FLUJO7":dbl, "fFLUJO4"=→"Flujo8." →"FLUJO8":dbl)  [unwired: 2 out]
            n117 = Cluster To Array(cluster=w256) -> (array=w278:dbl[])
            n118 = Build Array (concatenate)(w281, w278) -> (w280:dbl[][])
            n119 = local write "Array"(w280) -> ()
            n120 = global write "P2022 TB INCAR GLOBALES.vi" "Delta_T (C)"("Delta_T (C)") -> ()
            n121 = global write "P2022 TB INCAR GLOBALES.vi" "Delta_t (s)"("Delta_t (s)") -> ()
            n122 = global write "P2022 TB INCAR GLOBALES.vi" "Max_t (s)"("Max_t (s)") -> ()
            n123 = Transpose 2D Array(2D array=w280) -> (transposed array=w279:dbl[][])
            n124 = global read "P2022 TB INCAR GLOBALES.vi" "TEMPERATURA"() -> (→"TEMPERATURA":string)
            n125 = global read "P2022 TB INCAR GLOBALES.vi" "Arduino"() -> (w213:T1)
            n126 = global read "P2022 TB INCAR GLOBALES.vi" "PESO"() -> (→"PESO":string)
            n127 = Unbundle By Name(w213) -> ("Evalve"=→"Lvalve":bool, "EVflujo1"=→"Lflujo1":bool, "EVflujo2"=→"Lflujo2":bool, "EVflujo3"=→"Lflujo3":bool, "EVflujo4"=→"Lflujo4":bool)
            n128 = global write "P2022 TB INCAR GLOBALES.vi" "ModuloIN"("Modulo") -> ()
            n129 = Index Array(array=w279, index (row) #1=0 ("index (row)"), index (row) #2=10 ("index (row)"), index (row) #3=12 ("index (row)"), index (row) #4=14 ("index (row)"), index (row) #5=17 ("index (row)"), index (row) #6=16 ("index (row)"), index (row) #7=18 ("index (row)"), index (row) #8=0 ("index (row)"), index (row) #9=2 ("index (row)"), index (row) #10=4 ("index (row)"), index (row) #11=6 ("index (row)"), index (row) #12=8 ("index (row)"), index (row) #13=22 ("index (row)"), index (row) #14=24 ("index (row)"), index (row) #15=26 ("index (row)"), index (row) #16=28 ("index (row)")) -> (element #1=w203:dbl[], element #2=w260:dbl[], element #3=w259:dbl[], element #4=w258:dbl[], element #5=w215:dbl[], element #6=w216:dbl[], element #7=w257:dbl[], element #9=w234:dbl[], element #10=w235:dbl[], element #11=w236:dbl[], element #12=w237:dbl[], element #13=w198:dbl[], element #14=w197:dbl[], element #15=w196:dbl[], element #16=w195:dbl[])  [unwired: 16 in, 1 out]
            n130 = flat-sequence {
              tunnel: [w285] -> w253
              tunnel: w253 -> [w287]
              frame #0 {
                n131 = local read "mst0"() -> (w286:i32)
                n132 = Tick Count (ms)() -> (millisecond timer value=w285:u32)
                "mst1" <- w285
                n133 = Subtract(x=w285, y=w286) -> (x-y=→"Sampling(ms)":u32)
              }
              frame #1 {
                "mst0" <- w287
              }
            }
            n134 = Bundle(w203, w234) -> (w272:cluster{dbl[], dbl[]})  [unwired: 1 in]
            n135 = Bundle(w203, w235) -> (w271:cluster{dbl[], dbl[]})  [unwired: 1 in]
            n136 = Bundle(w203, w236) -> (w270:cluster{dbl[], dbl[]})  [unwired: 1 in]
            n137 = Bundle(w203, w237) -> (w269:cluster{dbl[], dbl[]})  [unwired: 1 in]
            n138 = Bundle(w203, w198) -> (w191:cluster{dbl[], dbl[]})  [unwired: 1 in]
            n139 = Bundle(w203, w197) -> (w192:cluster{dbl[], dbl[]})  [unwired: 1 in]
            n140 = Bundle(w203, w196) -> (w193:cluster{dbl[], dbl[]})  [unwired: 1 in]
            n141 = Bundle(w203, w195) -> (w194:cluster{dbl[], dbl[]})  [unwired: 1 in]
            n142 = global read "P2022 TB INCAR GLOBALES.vi" "PASOS"() -> (w188:string[])
            n143 = global read "P2022 TB INCAR GLOBALES.vi" "Arduino"() -> (→"ESTADO":T1)
            n144 = Bundle(w203, w260) -> (w276:cluster{dbl[], dbl[]})  [unwired: 1 in]
            n145 = Bundle(w203, w259) -> (w277:cluster{dbl[], dbl[]})  [unwired: 1 in]
            n146 = Bundle(w203, w258) -> (w267:cluster{dbl[], dbl[]})  [unwired: 1 in]
            n147 = Bundle(w203, w215) -> (w262:cluster{dbl[], dbl[]})  [unwired: 1 in]
            n148 = Bundle(w203, w216) -> (w261:cluster{dbl[], dbl[]})  [unwired: 1 in]
            n149 = Bundle(w203, w257) -> (w265:cluster{dbl[], dbl[]})  [unwired: 1 in]
            n150 = Bundle(w203, w215) -> (w264:cluster{dbl[], dbl[]})  [unwired: 1 in]
            n151 = Bundle(w203, w216) -> (w217:cluster{dbl[], dbl[]})  [unwired: 1 in]
            n152 = Bundle(w215, w257) -> (→"XYTemPes":cluster{dbl[], dbl[]})  [unwired: 1 in]
            n153 = local write "PASOS"(w188) -> ()
            n154 = Build Array(w272, w271, w270, w269, w191, w192, w193, w194) -> (→"XYFlows":cluster{dbl[], dbl[]}[])
            n155 = Build Array(w265, w264, w217) -> (→"XY Peso":cluster{dbl[], dbl[]}[])
            n156 = Build Array(w276, w277, w267, w262, w261) -> (→"XYTemp":cluster{dbl[], dbl[]}[])
          }
          frame "Upd Status" {
            n157 = Variant To Data(error in=w294, type=" ", Variant=w295) -> (data=→"Estado":string, error out=w293:errorcluster)
            n158 = global read "P2022 TB INCAR GLOBALES.vi" "PASOS"() -> (w289:string[])
            n159 = global read "P2022 TB INCAR GLOBALES.vi" "Pausa"() -> (w290:bool)
            n160 = local write "PASOS"(w289) -> ()
            n161 = property on="Pausa" class="Bool (strict)"("Blinking"=w290) -> ()  [unwired: 2 in, 2 out]
            n162 = global read "P2022 TB INCAR GLOBALES.vi" "PASOS"() -> (w288:string[])
            n163 = local write "PASOS"(w288) -> ()
          }
          frame "Upd Seq" {
            n164 = Variant To Data(error in=w302, type=0, Variant=w300) -> (data=w298:i32, error out=w301:errorcluster)
            n165 = Subtract(x=w298, y=4) -> (x-y=w299:i32)
            n166 = property on="Completa" class="LstBox (strict)"("Value (Signaling)"=w298) -> ()  [unwired: 2 in, 2 out]
            n167 = property on="Completa" class="LstBox (strict)"("Top Row"=w299) -> ()  [unwired: 2 in, 2 out]
            n168 = global read "P2022 TB INCAR GLOBALES.vi" "PASOS"() -> (w296:string[])
            n169 = local write "PASOS"(w296) -> ()
          }
        }
      }
    }
  }
  n170 = while {
    shift-right: [w309] -> w28
    shift-left: w23 -> [w311]
    shift-right: [w305] -> w27
    shift-left: w22 -> [w310]
    tunnel: w21 -> [w304]
    stop <- w307 stop-if-true
    n171 = Dequeue Element(queue=w311, error in (no error)=w310) -> (queue out=w309:refnum<queue>, element=w306:cluster{"Enum":T9, "Variant":variant}, error out=w308:errorcluster)  [unwired: 1 in, 1 out]
    n172 = case shown="No Error" w308 {
      selector: w308 -> [w315 w341]
      tunnel: [w313 _] -> w307
      tunnel: w306 -> [w317 _]
      tunnel: [w314 w341] -> w305
      tunnel: w304 -> [w312 _]
      frame No Error {
        n173 = Unbundle By Name(w317) -> ("Enum"=w316:T9)  [unwired: 1 out]
        n174 = case shown="\"Run Man\"" w316 {
          tunnel: w315 -> [w325 w329 w335 w339]
          tunnel: [w324 w328 w334 w338] -> w314
          tunnel: [FALSE FALSE FALSE TRUE] -> w313
          tunnel: w312 -> [w323 _ _ _]
          frame "Initialize", Default {
            n175 = call "P2022 TB INCAR_Initialize.vi"("error in (no error)"=w325, "User event"=w323) -> ("error out"=w324:errorcluster, "FLOWBUS_MassFlows"=w319:T12, "SERIAL_MassFlows"=w318:T12, "Comunicaciones"=w322:T5)  [unwired: 6 in]
            "Comunicaciones" <- w322
            n176 = global write "P2022 TB INCAR GLOBALES.vi" "Comunicaciones"(w322) -> ()
            n177 = global write "P2022 TB INCAR GLOBALES.vi" "serial_MassFlow"(w318) -> ()
            n178 = global write "P2022 TB INCAR GLOBALES.vi" "flowbus_MassFlow"(w319) -> ()
            n179 = Unbundle By Name(w318) -> ("Dispositivos"=→"SERIAL MassFlowDevs":T3)
            n180 = Unbundle By Name(w319) -> ("Dispositivos"=→"FLOWBUS MassFlowDevs":T3)
          }
          frame "Run Man" {
            # "P2018 TB INCAR_Run Manual"
            n181 = global read "P2022 TB INCAR GLOBALES.vi" "Comunicaciones"() -> (w327:T5)
            n182 = call "P2018 TB INCAR_Run Manual.vi"("Comunicaciones"=w327, "error in (no error)"=w329) -> ("error out"=w328:errorcluster)  [unwired: 9 in]
          }
          frame "Run Auto" {
            # "P2018 TB INCAR_Run Auto.vi\nvalvulas de seguridad MFCs"
            n183 = global read "P2022 TB INCAR GLOBALES.vi" "Comunicaciones"() -> (w332:T5)
            n184 = local read "Modulo"() -> (w331:u32)
            n185 = call "P2019 TB INCAR_Run Auto.vi"("ModuloIN"=w331, "error in (no error)"=w335, "Comunicaciones"=w332, "Secuencia"="Secuencia") -> ("error out"=w334:errorcluster)  [unwired: 7 in]
          }
          frame "Stop" {
            n186 = local read "Comunicaciones"() -> (w337:T5)
            n187 = call "P2018 TB INCAR_Shutdown.vi"("error in (no error)"=w339, "Comunicaciones"=w337) -> ("error out"=w338:errorcluster)  [unwired: 9 in]
          }
        }
      }
      frame Error {
      }
    }
  }
  n188 = Release Queue(queue=w28, error in (no error)=w27) -> (error out=w30:errorcluster)  [unwired: 1 in, 2 out]
  n189 = Unregister For Events(event registration refnum=w25, error in=w30) -> (error out=w31:errorcluster)
  n190 = Destroy User Event(user event=w21, error in=w31) -> (error out=w32:errorcluster)
  n191 = Merge Errors(w29, w32) -> (w19:errorcluster)
  n192 = flat-sequence {
    tunnel: w19 -> [w343]
    tunnel: [w343] -> w18
    frame #0 {
      n193 = Quit LabVIEW(quit? (T)=TRUE) -> ()
    }
  }
  "error out" <- w18
  "String2s" <- "AiR" ("String2")
  "String3s" <- "CO2" ("String3")
  "String4s" <- "N2" ("String4")
  "String1s" <- "H2O" ("String1")
  "String1f" <- "GAS1f" ("String1f")
  "String2f" <- "GAS2f" ("String2f")
  "String4f" <- "GAS4f" ("String4f")
  "String3f" <- "GAS3f" ("String3f")
  "PASOS" <- string[] [] ("PASOS")
